vi "command home.vi"(8 "error in (no error)":errorcluster, 11 "id":i32) -> (0 "error out":errorcluster, 3 "function return":i32)   [LabVIEW 2012, in "libximc.lvlib"]
doc: "result_t XIMC_API command_home (device_t id);"
uses:
  libximc.lvlib
  libximc.dll
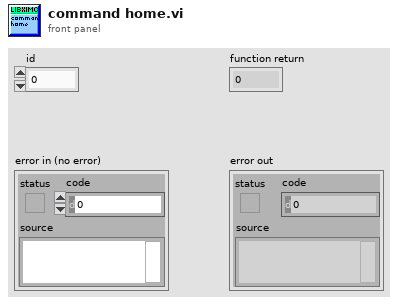
[diagram p1: front panel]
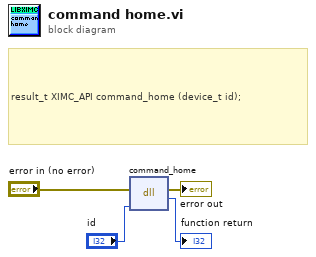
[diagram p0: block diagram]
diagram:
  # "result_t XIMC_API command_home (device_t id);"
  n1 = dll-call lib="C:/Users/Vasily/Att_examples/LabVIEW_example/libximc.*" fn="command_home"(error in="error in (no error)", "id"="id") -> (error out=→"error out":errorcluster, →"function return":i32)  [unwired: 3 in, 1 out]
